vi "fgt set Ttl Mode.vi"(8 "error in (no error)":errorcluster, 10 "mode":T1, 11 "TtlIndex":u32) -> (0 "error out":errorcluster)   [LabVIEW 2016, in "fgt_SDK.lvlib"]
doc: "Configure a specific TTL port (BNC ports) as input, output, rising or falling edge."
uses:
  fgt_SDK.lvlib
  TypeDefs/fgt_TTL_MODE.ctl
  dlls/fgt_SDK_32.dll
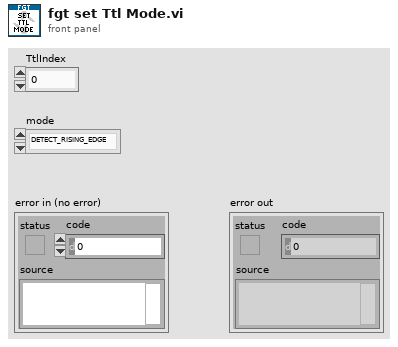
[diagram p1: front panel]
types:
  T1 = typedef "fgt_SDK.lvlib/fgt_TTL_MODE.ctl" = enum16{"DETECT_RISING_EDGE", "DETECT_FALLING_EDGE", "OUTPUT_PULSE_LOW", "OUTPUT_PULSE_HIGH"}
  T2 = typedef "fgt_SDK.lvlib/fgt_STATUS_INFO.ctl" = cluster{"InstrType":T3, "instrSN":u16, "errorCode":u8, "infoCode":u8, "detail":string}
  T3 = typedef "fgt_SDK.lvlib/fgt_INSTRUMENT_TYPE.ctl" = enum32{"None", "MFCS", "MFCS_EZ", "FRP", "LineUP"}
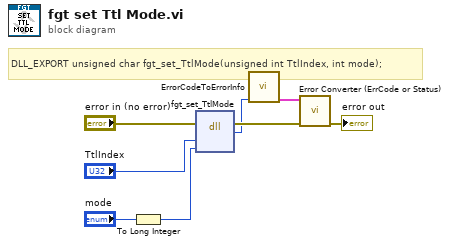
[diagram p0: block diagram]
diagram:
  # "DLL_EXPORT unsigned char fgt_set_TtlMode(unsigned int TtlIndex, int mode);"
  n1 = To Long Integer(number="mode") -> (32bit integer=w3:i32)
  n2 = dll-call lib="PTH2Zabs D\nMes DocumentsDéveloppementFluigentSDKsfgt-sdk-labviewdllsfgt_SDK_*.*" fn="fgt_set_TtlMode"(error in="error in (no error)", "TtlIndex"="TtlIndex", "mode"=w3) -> (error out=w5:errorcluster, "return type"=w2:u8)  [unwired: 4 in, 1 out]
  n3 = call "ErrorCodeToErrorInfo.vi"("return type"=w2) -> ("StatusInfo"=w1:T2)  [unwired: 10 in]
  n4 = call "Error Converter (ErrCode or Status).vi"("error in (no error)"=w5, "StatusInfo"=w1) -> ("error out"=→"error out":errorcluster)  [unwired: 9 in]
